vi "operate.vi"(8 "error in (no error)":errorcluster, 11 "reference in":refnum<class "GUI Controller.lvclass">) -> (0 "error out":errorcluster, 3 "reference out":refnum<class "GUI Controller.lvclass">)   [LabVIEW 2015, in "GUI Controller.lvclass"]
uses:
  GUI Controller.lvclass
  addNewFile.ctl
  myControl/calculationButton.ctl
  APP/subject_class/resultsType.ctl
  state.ctl
  APP/subject_class/phase.ctl
  Project Panels_class/Project Panels.lvclass
  SYS/File Controller_llb/File Controller.lvclass
  SYS/Subject Controller_llb/Subject Controller.lvclass
  APP/subject_class/subject.lvclass
panel:
  out "Title":string
  out "Duration (s)":dbl[](array[numeric]) format="%#.2g"
  out "Amplitude (L/min)":dbl[](array[numeric]) format="%#.2g"
  in  "Select type of results:":T1
  in  "Calculate":T2
  in  "Width (s):":i32
  in  "Threshold (L/min):":dbl format="%#.2g"
  out "Ventilation":cluster{"time_exer":dbl[], "Ve_exer":dbl[]}(graph)
  in  "Select Patient:":u16(ring) items=["Test1.xls"]
  in  "AddNewFile":T3
  out "StatusBar":string
  in  "Stop Button":bool
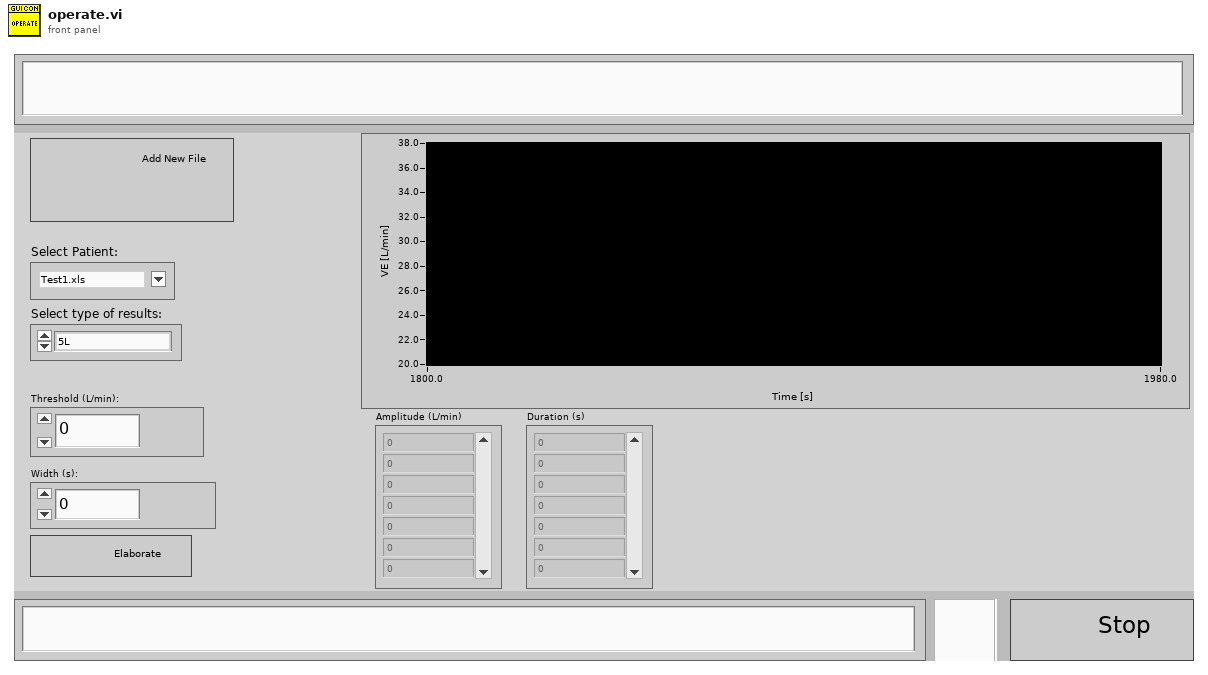
[diagram p1: front panel]
types:
  T1 = typedef "subject.lvclass/resultsType.ctl" = enum16{"5L", "15%", "User Selection"}
  T2 = typedef "calculationButton.ctl" = bool
  T3 = typedef "GUI Controller.lvclass/addNewFile.ctl" = bool
  T4 = typedef "GUI Controller.lvclass/state.ctl" = enum16{"initiate", "AddNewFile", "ElaborateData", "waitEvent", "ChangeSubject", "stop"}
  T5 = enum32{"Invalid", "Standard", "Closed", "Hidden", "Minimized", "Maximized"}
  T6 = typedef "subject.lvclass/phase.ctl" = enum16{"warmUp", "userSelection", "Exercise"}
  T7 = typedef "GUI Controller.lvclass/ObjectAttributesRef.ctl" = refnum<data-value>
  T8 = typedef "GUI Controller.lvclass/ObjectAttributes.ctl" = cluster{"MyAttribute":dbl, "state":T4, "project_panels_ref":refnum<class "Project Panels.lvclass">, "file_controller_ref":refnum<class "File Controller.lvclass">, "subject_controller_ref":refnum<class "Subject Controller.lvclass">}
  T9 = enum8{"Enabled", "Disabled", "Disabled and Grayed Out"}
  T10 = cluster{"Ve_warm":dbl[], "time_warm":dbl[], "name":string, "phase":dbl[], "VCO2":dbl[], "VO2":dbl[], "PetCO2":dbl[], "RQ":dbl[], "HR":dbl[], "Ve_warm_inter":dbl[], "time_warm_inter":dbl[], "Ve_exer":dbl[], "time_exer":dbl[], "Ve_exer_inter":dbl[], "time_exer_inter":dbl[], "Ve":dbl[], "time":dbl[]}
  T11 = cluster{"EOV":bool, "osci_amplitude":dbl[], "osci_width":dbl[], "peak_location":dbl[], "threshold":dbl, "width":i32}
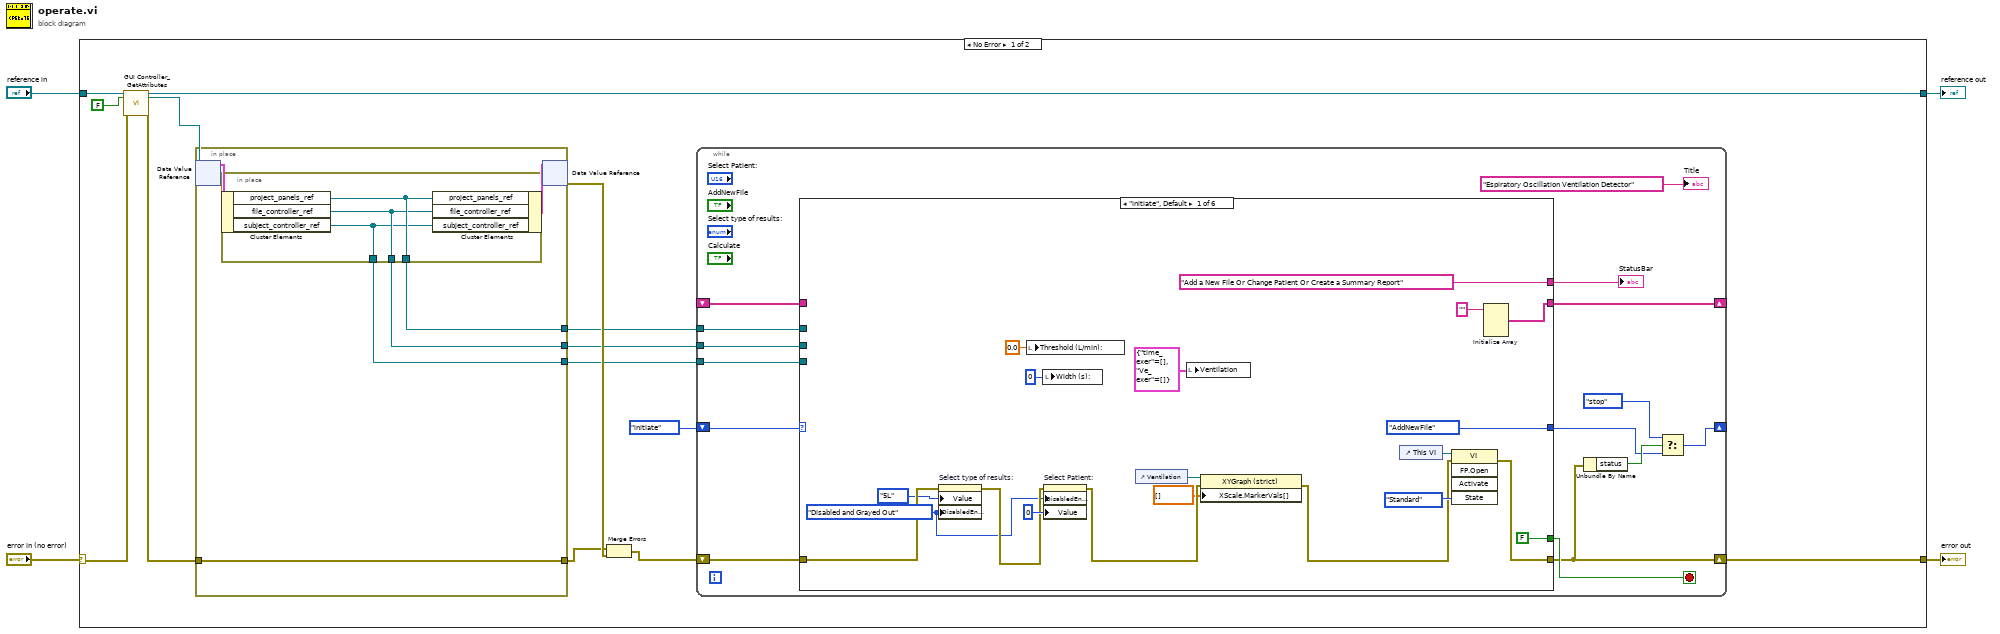
[diagram p0: block diagram]
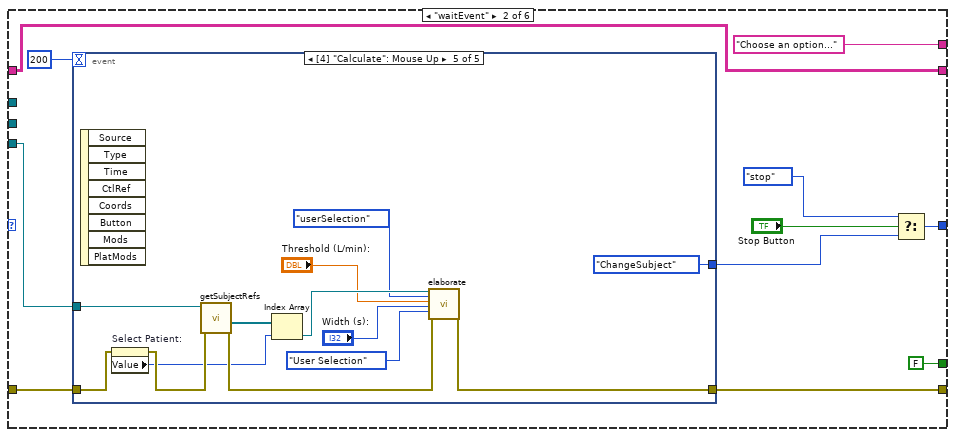
[diagram p2: hidden frame]
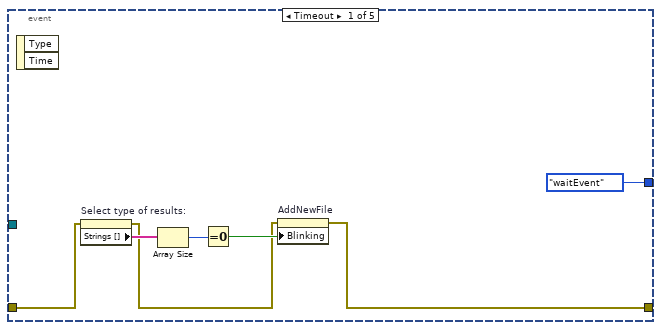
[diagram p3: hidden frame]
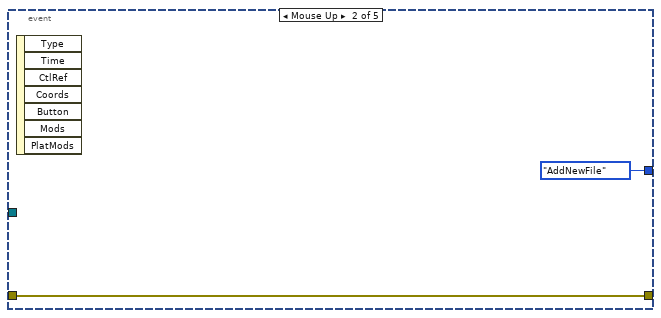
[diagram p4: hidden frame]
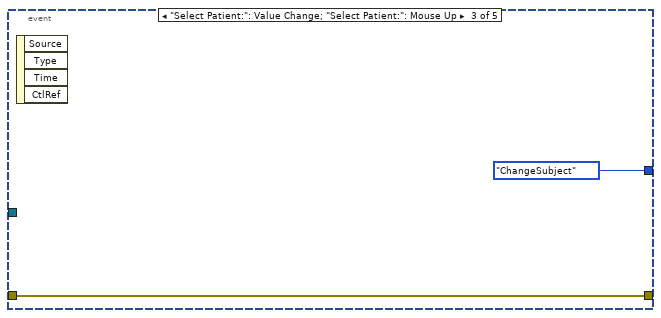
[diagram p5: hidden frame]
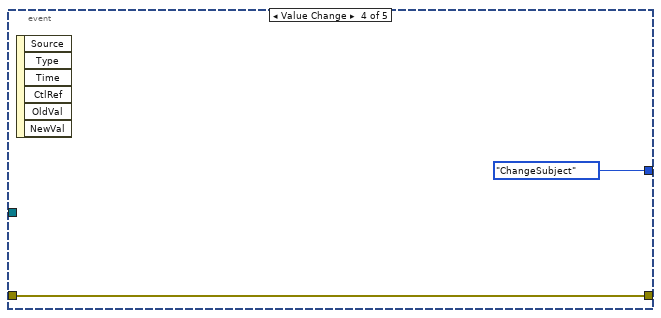
[diagram p6: hidden frame]
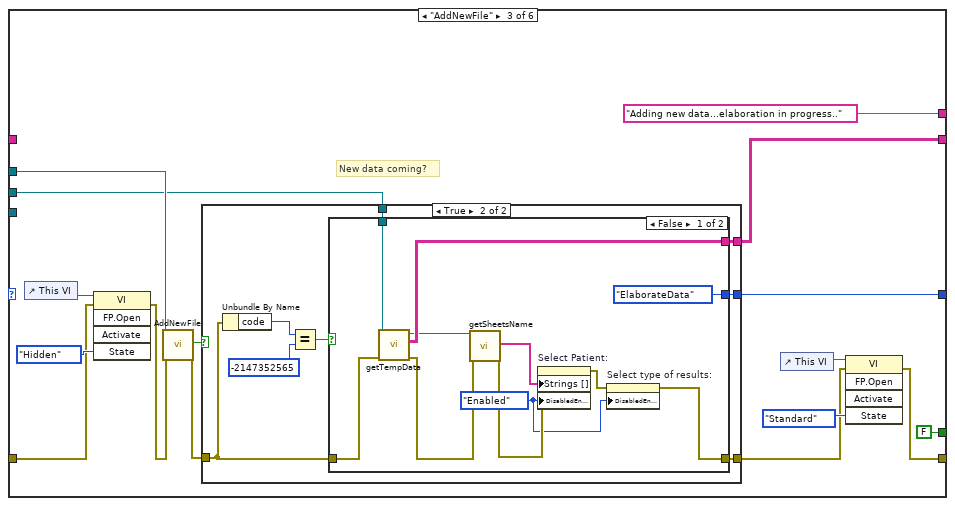
[diagram p7: hidden frame]
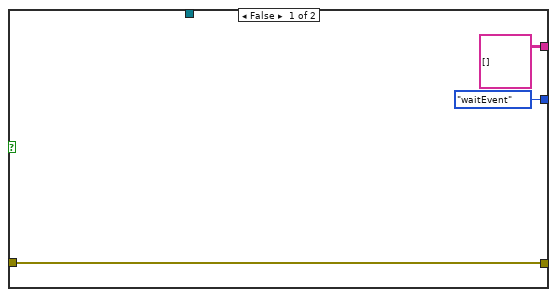
[diagram p8: hidden frame]
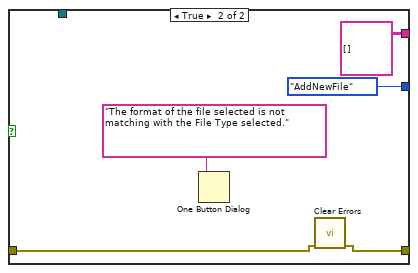
[diagram p9: hidden frame]
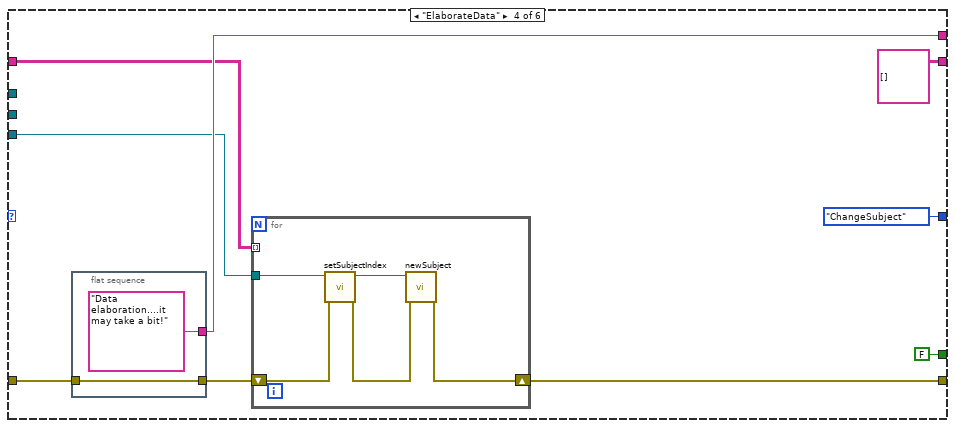
[diagram p10: hidden frame]
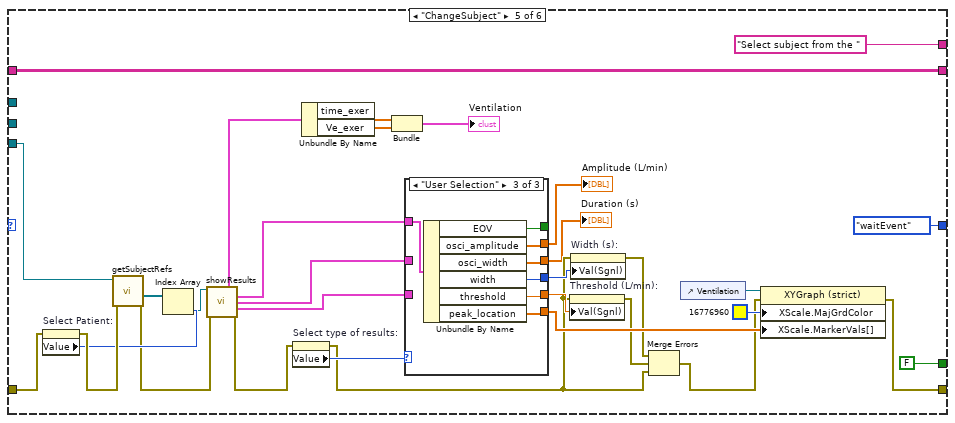
[diagram p11: hidden frame]
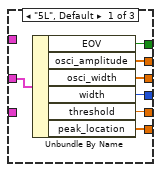
[diagram p12: hidden frame]
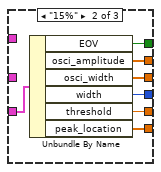
[diagram p13: hidden frame]
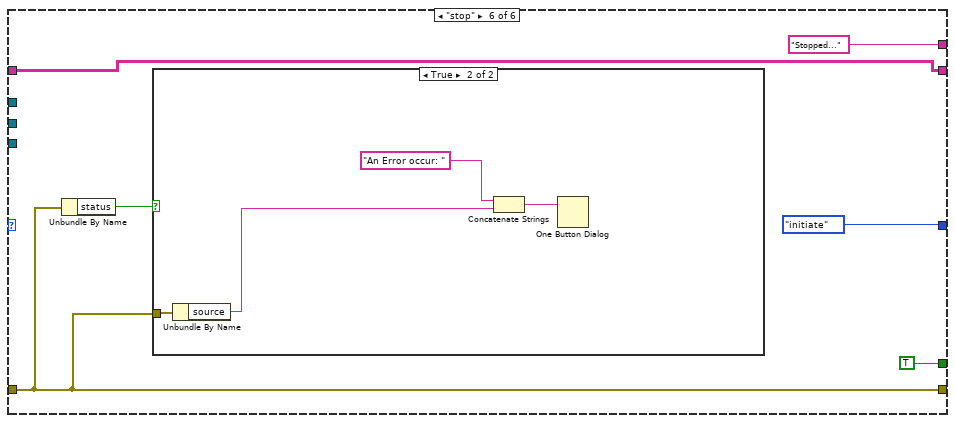
[diagram p14: hidden frame]
diagram:
  n1 = case shown="No Error" "error in (no error)" {
    selector: "error in (no error)" -> [w14 w223]
    tunnel: [w8 w223] -> w3
    tunnel: [w12 w222] -> w1
    tunnel: "reference in" -> [w16 w222]
    frame No Error {
      n2 = call "GUI Controller_GetAttributes.vi"("reference in"=w16, "return data? (T)"=FALSE, "error in (no error)"=w14) -> ("reference out"=w12:refnum<class "GUI Controller.lvclass">, "attributes ref"=w11:T7, "error out"=w13:errorcluster)  [unwired: 13 in, 1 out]
      n3 = in-place {
        in-place-border: w13 -> [w216]
        in-place-border: [w216] -> w17
        in-place-border: [w215] -> w7
        in-place-border: [w214] -> w6
        in-place-border: [w213] -> w5
        n4 = in-place-dvr #1(w11) -> (w217:T8)  [unwired: 1 out]
        n5 = in-place {
          in-place-border: [w221] -> w214
          in-place-border: [w220] -> w215
          in-place-border: [w219] -> w213
          n6 = in-place-cluster #2(w217) -> ("project_panels_ref"=w221:refnum<class "Project Panels.lvclass">, "file_controller_ref"=w220:refnum<class "File Controller.lvclass">, "subject_controller_ref"=w219:refnum<class "Subject Controller.lvclass">)
          n7 = in-place-cluster #2("project_panels_ref"=w221, "file_controller_ref"=w220, "subject_controller_ref"=w219) -> (w218:T8)
        }
        n8 = in-place-dvr #1(w218) -> (w18:errorcluster)  [unwired: 1 out]
      }
      n9 = Merge Errors(w17, w18) -> (w10:errorcluster)
      n10 = while {
        shift-right: [w26] -> _
        shift-left: state."initiate" ("state") -> [w32]
        shift-right: [w28] -> w8
        shift-left: w10 -> [w33]
        tunnel: w7 -> [w23]
        tunnel: w6 -> [w22]
        tunnel: w5 -> [w21]
        shift-right: [w20] -> _
        shift-left: _ -> [w19]
        stop <- w29 stop-if-true
        n11 = case shown="\"initiate\", Default" w32 {
          tunnel: w33 -> [w44 w59 w102 w141 w178 w205]
          tunnel: [w49 w58 w94 w137 w170 w205] -> w28
          tunnel: [state."AddNewFile" ("state") w61 w93 state."ChangeSubject" ("state") state."waitEvent" ("f") state."initiate" ("state")] -> w25
          tunnel: ["Add a New File Or Change Patient Or Create a Summary Report" ("Title") "Choose an option..." ("Title") "Adding new data...elaboration in progress.." ("Title") w140 "Select subject from the " ("Title") "Stopped..." ("Title")] -> w31
          tunnel: [FALSE FALSE FALSE FALSE FALSE TRUE] -> w29
          tunnel: w23 -> [_ _ w99 _ _ _]
          tunnel: w22 -> [_ _ w101 _ _ _]
          tunnel: w21 -> [_ w54 _ w136 w175 _]
          tunnel: [w46 w55 w92 string[][][] [] ("data") w177 w203] -> w20
          tunnel: w19 -> [_ w55 _ w135 w177 w203]
          frame "initiate", Default {
            w37 = T9."Disabled and Grayed Out" ("Disabled")
            n12 = property on="Select type of results:" class="Enum (strict)"(error in=w44, "Value"=resultsType."5L" ("Select type of results:"), "DisabledEnum"=w37) -> (error out=w43:errorcluster)  [unwired: 1 in, 1 out]
            n13 = local write "Threshold (L/min):"(0.0 ("Threshold (L/min):")) -> ()
            n14 = local write "Width (s):"(0 ("Width (s):")) -> ()
            n15 = property on="Select Patient:" class="Ring (strict)"(error in=w43, "DisabledEnum"=w37, "Value"=0) -> (error out=w36:errorcluster)  [unwired: 1 in, 1 out]
            n16 = control-ref of="Ventilation"() -> (w38:refnum<vi>)
            n17 = local write "Ventilation"(cluster{"time_exer":dbl[], "Ve_exer":dbl[]} {"time_exer"=[], "Ve_exer"=[]} ("Ventilation")) -> ()
            n18 = property on="Property Node" class="XYGraph (strict)"(reference=w38, error in=w36, "XScale.MarkerVals[]"=dbl[] [] ("X Scale.Marker Values[]")) -> (error out=w35:errorcluster)  [unwired: 1 out]
            n19 = control-ref of="This VI"() -> (w50:refnum<vi>)
            n20 = invoke class="VI" method="FP.Open"(reference=w50, error in=w35, "State"=T5."Standard") -> (error out=w49:errorcluster)  [unwired: 2 in, 4 out]
            n21 = Initialize Array("") -> (w46:string[][][])  [unwired: 3 in]
          }
          frame "waitEvent" {
            n22 = event shown="[4] \"Calculate\": Mouse Up" {
              selector: _ -> [_ _ _ _ _]
              dyn-events: _ -> [_ _ _ _ _]
              timeout: 200 -> [_ _ _ _ _]
              tunnel: w59 -> [w67 w72 w74 w76 w88]
              tunnel: [w65 w72 w74 w76 w89] -> w58
              tunnel: [state."waitEvent" ("f") state."AddNewFile" ("f") state."ChangeSubject" ("f") state."ChangeSubject" ("f") state."ChangeSubject" ("f")] -> w56
              tunnel: w54 -> [_ _ _ _ w85]
              event Timeout {
                n23 = event-data() -> ()  [unwired: 1 in, 2 out]
                n24 = property on="Select type of results:" class="Enum (strict)"(error in=w67) -> (error out=w66:errorcluster, "Strings []"=w70:string[])  [unwired: 1 in, 1 out]
                n25 = Array Size(array=w70) -> (size(s)=w69:i32)
                n26 = Equal To 0?(x=w69) -> (x = 0?=w68:bool)
                n27 = property on="AddNewFile" class="Bool (strict)"(error in=w66, "Blinking"=w68) -> (error out=w65:errorcluster)  [unwired: 1 in, 1 out]
              }
              event Mouse Up {
                n28 = event-data() -> ()  [unwired: 1 in, 7 out]
              }
              event "Select Patient:": Value Change; "Select Patient:": Mouse Up {
                n29 = event-data() -> ()  [unwired: 1 in, 4 out]
              }
              event Value Change {
                n30 = event-data() -> ()  [unwired: 1 in, 6 out]
              }
              event Mouse Up {
                n31 = event-data() -> ()  [unwired: 1 in, 8 out]
                n32 = property on="Select Patient:" class="Ring (strict)"(error in=w88) -> (error out=w87:errorcluster, "Value"=w83:u16)  [unwired: 1 in, 1 out]
                n33 = call "getSubjectRefs.vi"("error in (no error)"=w87, "reference in"=w85) -> ("error out"=w86:errorcluster, "subject_refs"=w84:refnum<class "subject.lvclass">[])  [unwired: 7 in, 1 out]
                n34 = Index Array(array=w84, index=w83) -> (element=w82:refnum<class "subject.lvclass">)
                n35 = call "elaborate.vi"("reference in"=w82, "phase"=phase."userSelection", "threshold"="Threshold (L/min):", "Width"="Width (s):", "resultsType"=resultsType."User Selection", "error in (no error)"=w86) -> ("error out"=w89:errorcluster)  [unwired: 12 in, 1 out]
              }
            }
            n36 = Select(t=state."stop" ("state"), s="Stop Button", f=w56) -> (s? t:f=w61:T4)
          }
          frame "AddNewFile" {
            # "New data coming?"
            n37 = control-ref of="This VI"() -> (w104:refnum<vi>)
            n38 = invoke class="VI" method="FP.Open"(reference=w104, error in=w102, "State"=T5."Hidden") -> (error out=w100:errorcluster)  [unwired: 2 in, 4 out]
            n39 = call "AddNewFile.vi"("reference in"=w101, "error in (no error)"=w100) -> ("newData?"=w91:bool, "error out"=w98:errorcluster)  [unwired: 15 in, 1 out]
            n40 = case shown="True" w91 {
              tunnel: w99 -> [_ w117]
              tunnel: w98 -> [w109 w116]
              tunnel: [w109 w112] -> w95
              tunnel: [state."waitEvent" ("state") w111] -> w93
              tunnel: [string[][][] [] ("data") w110] -> w92
              frame False {
              }
              frame True {
                n41 = Unbundle By Name(w116) -> ("code"=w115:i32)
                n42 = Equal?(x=w115, y=-2147352565) -> (x = y?=w113:bool)
                n43 = case shown="False" w113 {
                  tunnel: w116 -> [w128 w132]
                  tunnel: w117 -> [w127 _]
                  tunnel: [w126 string[][][] [] ("data")] -> w110
                  tunnel: [w119 w131] -> w112
                  tunnel: [state."ElaborateData" ("state") state."AddNewFile" ("state")] -> w111
                  frame False {
                    w118 = T9."Enabled" ("Disabled")
                    n44 = call "getTempData.vi"("error in (no error)"=w128, "reference in"=w127) -> ("error out"=w124:errorcluster, "temp_data"=w126:string[][][], "reference out"=w125:refnum<class "File Controller.lvclass">)  [unwired: 7 in]
                    n45 = call "getSheetsName.vi"("reference in"=w125, "error in (no error)"=w124) -> ("sheetName"=w123:string[], "error out"=w122:errorcluster)  [unwired: 15 in, 1 out]
                    n46 = property on="Select Patient:" class="Ring (strict)"(error in=w122, "Strings []"=w123, "DisabledEnum"=w118) -> (error out=w120:errorcluster)  [unwired: 1 in, 1 out]
                    n47 = property on="Select type of results:" class="Enum (strict)"(error in=w120, "DisabledEnum"=w118) -> (error out=w119:errorcluster)  [unwired: 1 in, 1 out]
                  }
                  frame True {
                    n48 = One Button Dialog(message="The format of the file selected is not matching with the File Type selected.") -> ()  [unwired: 1 in, 1 out]
                    n49 = call <vilib>:"Clear Errors.vi"("error in (no error)"=w132) -> ("error out"=w131:errorcluster)  [unwired: 5 in, 1 out]
                  }
                }
              }
            }
            n50 = control-ref of="This VI"() -> (w96:refnum<vi>)
            n51 = invoke class="VI" method="FP.Open"(reference=w96, error in=w95, "State"=T5."Standard") -> (error out=w94:errorcluster)  [unwired: 2 in, 4 out]
          }
          frame "ElaborateData" {
            n52 = flat-sequence {
              tunnel: w141 -> [w149]
              tunnel: [w149] -> w138
              tunnel: ["Data elaboration....it may take a bit!"] -> w140
              frame #0 {
              }
            }
            n53 = for {
              shift-right: [w143] -> w137
              shift-left: w138 -> [w147]
              tunnel: w135 -> [_] mode=indexing
              tunnel: w136 -> [w146]
              n54 = call "setSubjectIndex.vi"("error in (no error)"=w147, "reference in"=w146) -> ("error out"=w145:errorcluster, "reference out"=w144:refnum<class "Subject Controller.lvclass">)  [unwired: 8 in]
              n55 = call "newSubject.vi"("error in (no error)"=w145, "reference in"=w144) -> ("error out"=w143:errorcluster)  [unwired: 8 in, 1 out]
            }
          }
          frame "ChangeSubject" {
            n56 = property on="Select Patient:" class="Ring (strict)"(error in=w178) -> (error out=w176:errorcluster, "Value"=w173:u16)  [unwired: 1 in, 1 out]
            n57 = call "getSubjectRefs.vi"("error in (no error)"=w176, "reference in"=w175) -> ("error out"=w171:errorcluster, "subject_refs"=w174:refnum<class "subject.lvclass">[])  [unwired: 7 in, 1 out]
            n58 = Index Array(array=w174, index=w173) -> (element=w172:refnum<class "subject.lvclass">)
            n59 = call "showResults.vi"("reference in"=w172, "error in (no error)"=w171) -> ("data"=w162:T10, "results_user_selection"=w161:T11, "results_5l"=w160:T11, "results_15percent"=w159:T11, "error out"=w164:errorcluster)  [unwired: 7 in, 2 out]
            n60 = property on="Select type of results:" class="Enum (strict)"(error in=w164) -> (error out=w153:errorcluster, "Value"=w163:T1)  [unwired: 1 in, 1 out]
            n61 = Unbundle By Name(w162) -> ("time_exer"=w167:dbl[], "Ve_exer"=w166:dbl[])
            n62 = Bundle("time_exer"=w167, "Ve_exer"=w166) -> (→"Ventilation":cluster{"time_exer":dbl[], "Ve_exer":dbl[]})  [unwired: 1 in]
            n63 = case shown="\"User Selection\"" w163 {
              tunnel: w161 -> [_ _ w196]
              tunnel: w160 -> [w182 _ _]
              tunnel: w159 -> [_ w195 _]
              tunnel: [w184 w194 w197] -> w158
              tunnel: [w185 w193 w198] -> w156
              tunnel: [w186 w192 w199] -> w157
              tunnel: [w188 w191 w201] -> w151
              tunnel: [w187 w190 w200] -> w150
              tunnel: [w183 w189 w202] -> _
              frame "5L", Default {
                n64 = Unbundle By Name(w182) -> ("EOV"=w183:bool, "osci_amplitude"=w188:dbl[], "osci_width"=w187:dbl[], "width"=w186:i32, "threshold"=w185:dbl, "peak_location"=w184:dbl[])
              }
              frame "15%" {
                n65 = Unbundle By Name(w195) -> ("EOV"=w189:bool, "osci_amplitude"=w191:dbl[], "osci_width"=w190:dbl[], "width"=w192:i32, "threshold"=w193:dbl, "peak_location"=w194:dbl[])
              }
              frame "User Selection" {
                n66 = Unbundle By Name(w196) -> ("EOV"=w202:bool, "osci_amplitude"=w201:dbl[], "osci_width"=w200:dbl[], "width"=w199:i32, "threshold"=w198:dbl, "peak_location"=w197:dbl[])
              }
            }
            "Amplitude (L/min)" <- w151
            "Duration (s)" <- w150
            n67 = property on="Threshold (L/min):" class="DigNum (strict)"(error in=w153, "Val(Sgnl)"=w156) -> (error out=w154:errorcluster)  [unwired: 1 in, 1 out]
            n68 = property on="Width (s):" class="DigNum (strict)"(error in=w153, "Val(Sgnl)"=w157) -> (error out=w155:errorcluster)  [unwired: 1 in, 1 out]
            n69 = Merge Errors(w155, w154, w153) -> (w152:errorcluster)
            n70 = control-ref of="Ventilation"() -> (w168:refnum<vi>)
            n71 = property on="Property Node" class="XYGraph (strict)"(reference=w168, error in=w152, "XScale.MajGrdColor"=u32 16776960 ("Color Box"), "XScale.MarkerVals[]"=w158) -> (error out=w170:errorcluster)  [unwired: 1 out]
          }
          frame "stop" {
            n72 = Unbundle By Name(w205) -> ("status"=w204:bool)
            n73 = case shown="True" w204 {
              tunnel: w205 -> [_ w210]
              frame False {
              }
              frame True {
                n74 = Unbundle By Name(w210) -> ("source"=w209:string)
                n75 = Concatenate Strings("An Error occur: " ("message"), w209) -> (w212:string)
                n76 = One Button Dialog(message=w212) -> ()  [unwired: 1 in, 1 out]
              }
            }
          }
        }
        "StatusBar" <- w31
        n77 = Unbundle By Name(w28) -> ("status"=w27:bool)
        n78 = Select(t=state."stop", s=w27, f=w25) -> (s? t:f=w26:T4)
        "Title" <- "Espiratory Oscillation Ventilation Detector" ("Title")
      }
    }
    frame Error {
    }
  }
  "error out" <- w3
  "reference out" <- w1
